vi "posicion.vi"(11 "a0":dbl) -> (3 "Real Matrix":T1)   [LabVIEW 2018]
uses:
  <vilib>/Analysis/Matrix/Datatypes/RealMatrix.ctl
  <vilib>/Analysis/Matrix/NI_Matrix.lvlib
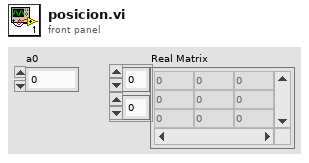
[diagram p1: front panel]
types:
  T1 = typedef "NI_Matrix.lvlib/RealMatrix.ctl" = dbl[][]
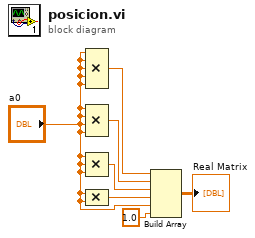
[diagram p0: block diagram]
diagram:
  n1 = Compound Arithmetic op=MULTIPLY("a0", "a0", "a0", "a0", "a0") -> (w1:dbl)
  n2 = Compound Arithmetic op=MULTIPLY("a0", "a0", "a0", "a0") -> (w2:dbl)
  n3 = Compound Arithmetic op=MULTIPLY("a0", "a0", "a0") -> (w3:dbl)
  n4 = Compound Arithmetic op=MULTIPLY("a0", "a0") -> (w4:dbl)
  n5 = Build Array(w1, w2, w3, w4, "a0", 1.0) -> (→"Real Matrix":T1)
